vi "FPGA_driver.vi"() -> ()   [LabVIEW 2019]
uses:
  <vilib>/Platform/TimedLoop/XDataNode/timing_clust.ctl
  <vilib>/Platform/TimedLoop/XDataNode/nitl_modes.ctl
  <vilib>/Platform/TimedLoop/XDataNode/wakeup.ctl
  <vilib>/rvi/Emulation/niFpgaGetClockAttributes.vi
  <vilib>/rvi/Emulation/niFpgaSctlEmulationGetInTimedLoop.vi
  <vilib>/rvi/Emulation/niFpgaEmulationReportErrorSimple.vi
  <vilib>/rvi/Emulation/niFpgaProcessEmulError.vi
  <vilib>/rvi/Emulation/niFpgaCriticalErrorInLSC.vi
  <vilib>/rvi/eio/common/nirviEmuTemplateMethod_errors.vi
  <vilib>/rvi/Analysis/common/FxpNativeNode/niFpgaFxpNative.xnode
  <vilib>/eio/EIONode/EIONode.xnode
  <vilib>/platform/TimedLoop/XDataNode/XDataNode.xnode
  <vilib>/Platform/TimedLoop/XDataNode/XDNodeRunTimeDep.lvlib
panel:
  out "Feed Reset":bool
  out "Steer Reset":bool
  in  "Num_cycle_on":u32
  in  "enable?":bool
  out "Encoder Position 2":i16
  in  "Encoder Reload Value 2":i16
  out "clk/pulse":i32
  out "Velocity\nValid?":bool
  in  "Position Ref.":i32
  in  "Num Clocks\nper Period":u32=400000
  in  "Velocity \nLimit":i32=10
  in  "Position Loop\nPeriod (ms)":u32=10
  out "Encoder Position":i16
  in  "Encoder Reload Value":i16
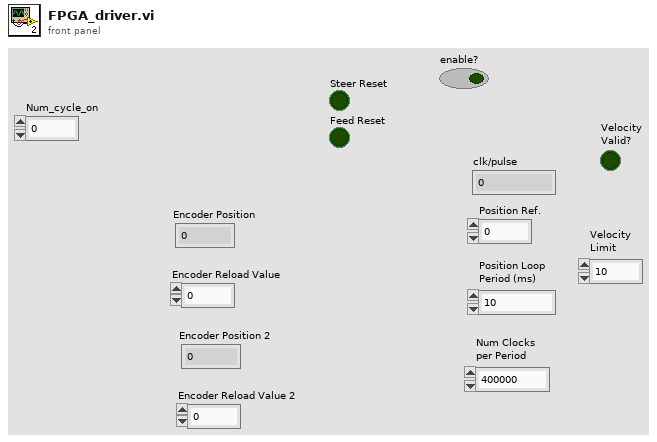
[diagram p1: front panel]
types:
  T1 = typedef "XDNodeRunTimeDep.lvlib/timing_clust.ctl" = cluster{"Expected End [f-1]":u64, "Actual End [f-1]":u64, "Finished Late? [f-1]":bool, "Expected End [i-1]":u64, "Actual End [i-1]":u64, "Finished Late? [i-1]":bool, "Expected Start [i]":u64, "Actual Start [i]":u64, "Expected Start [f]":u64, "Actual Start [f]":u64, "Source Name":string, "Structure Name":string, "Period":i64, "Deadline":i64, "Offset":i64, "Start":i64, "Priority":i32, "Timeout":i32, "Mode":T2, "Wakeup Reason":T3, "Error":errorcluster, "Source Type":string, "Secondary Source Type":string, "Global End Time":u64, "Global Start Time":u64, "Frame Duration":u64, "Iteration Duration":u64, "Assigned CPU":i32, "I/O Scan Engine Mode":u32}
  T2 = typedef "XDNodeRunTimeDep.lvlib/nitl_modes.ctl" = enum32{"No Change", "Process missed periods, maintain original phase", "Discard missed periods, maintain original phase", "Process missed periods, ignore original phase", "Discard missed periods, ignore original phase"}
  T3 = typedef "XDNodeRunTimeDep.lvlib/wakeup.ctl" = enum32{"Normal", "Aborted", "Asynchronous wakeup", "Timing source error", "Timed loop error", "Timeout"}
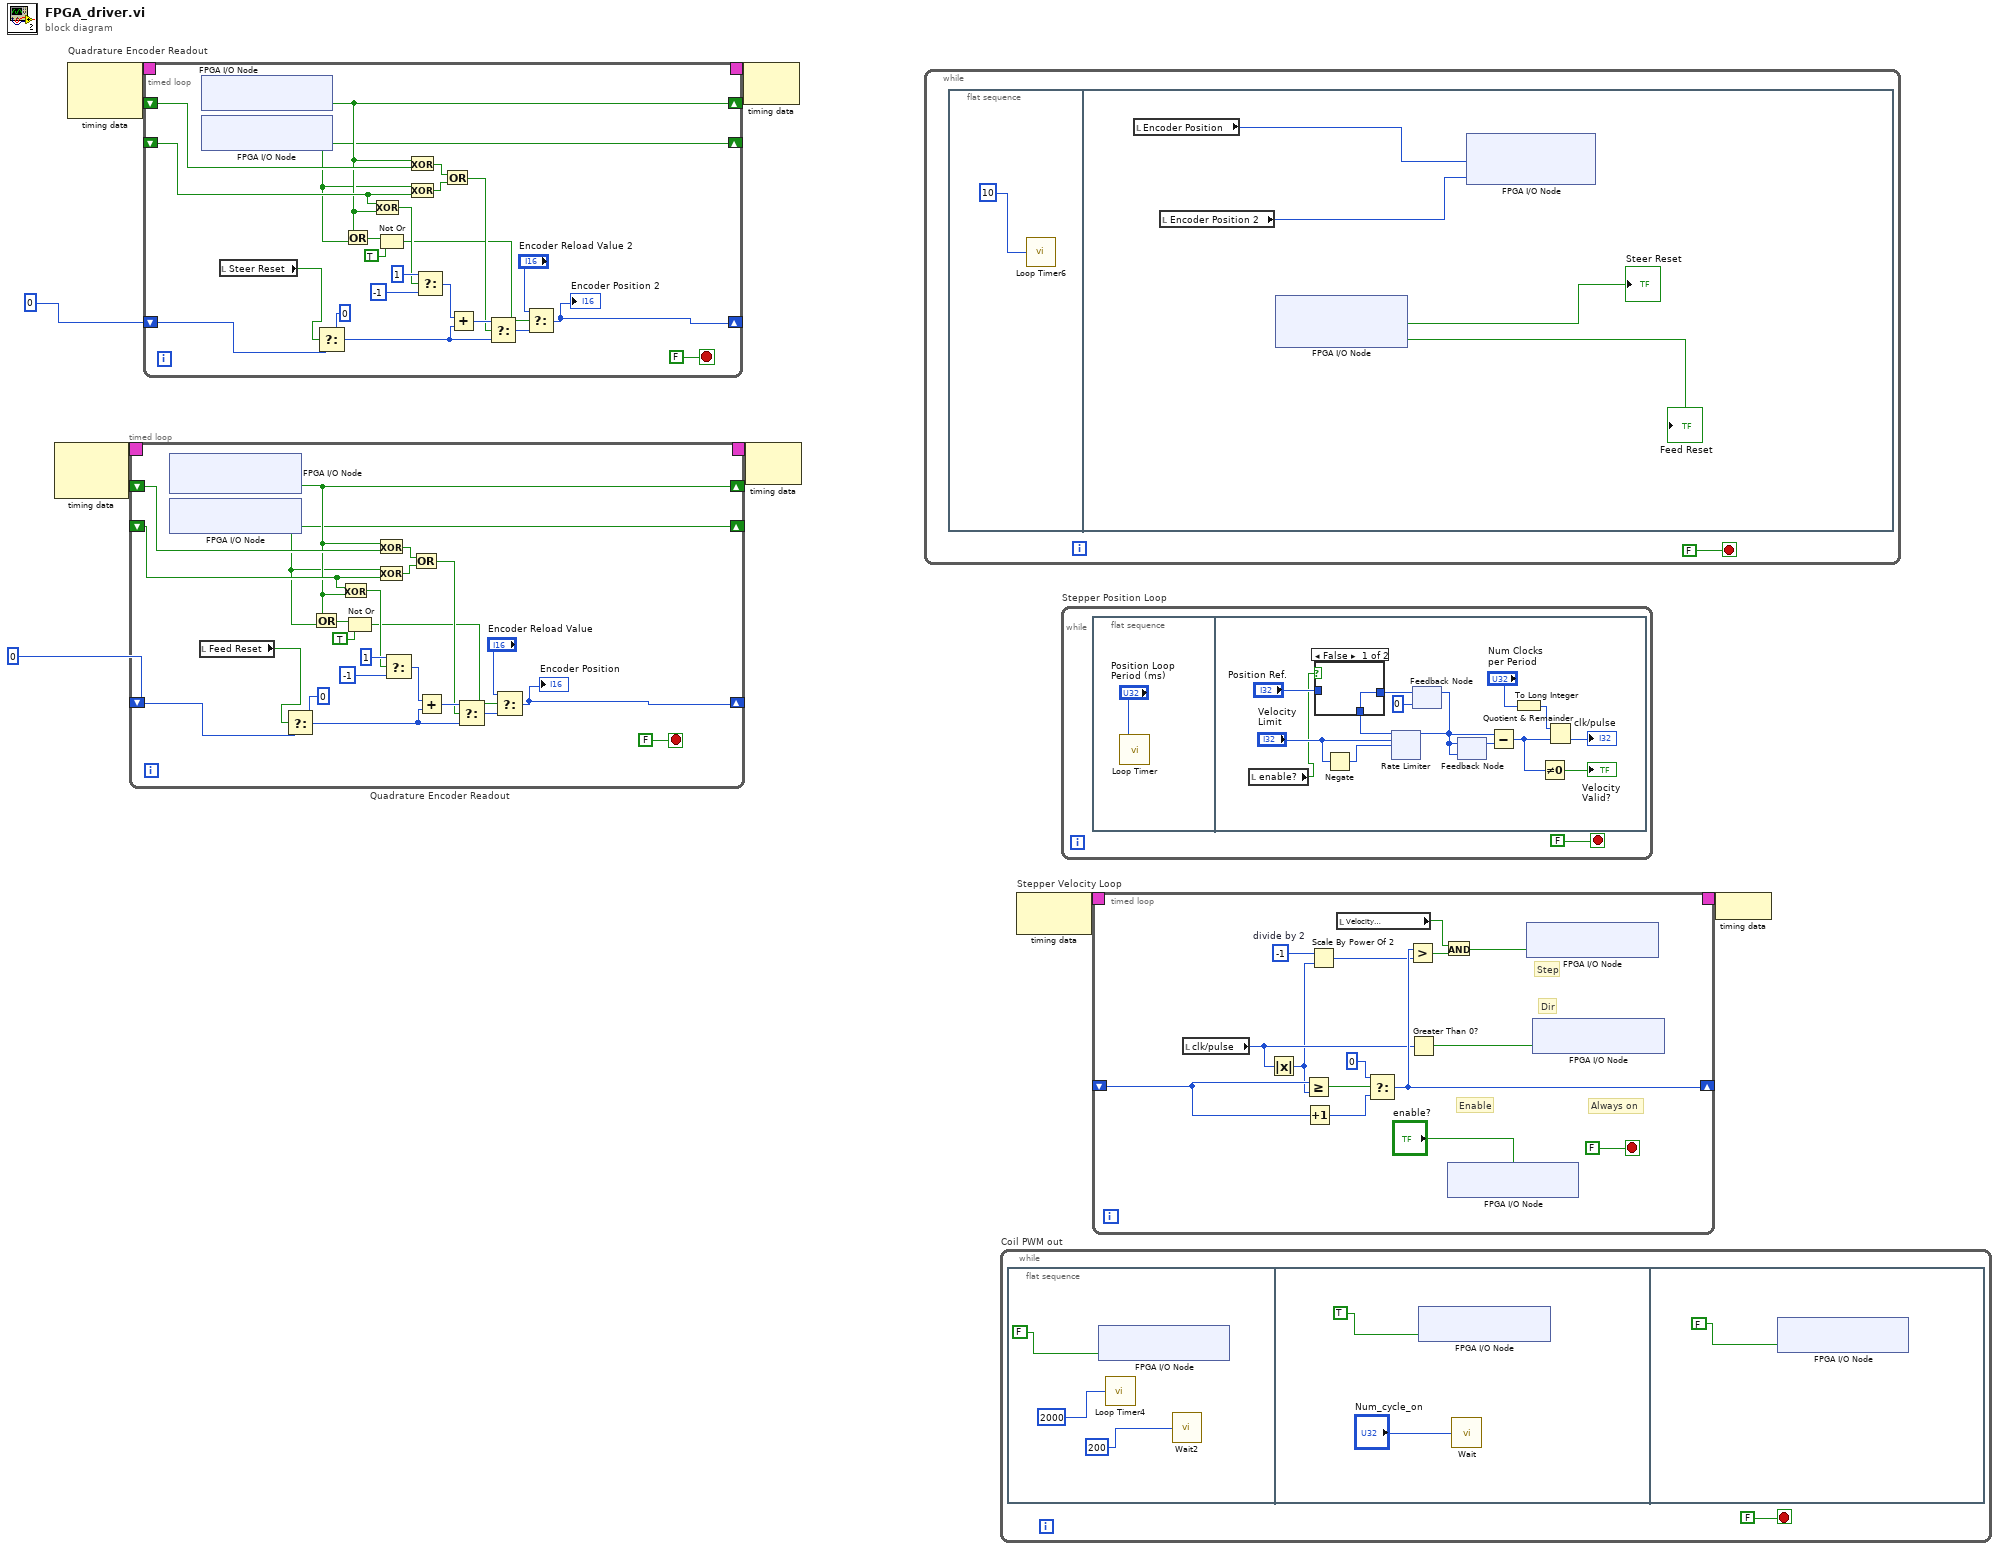
[diagram p0: block diagram]
diagram:
  n1 = node-c288() -> (w8:T1)  [unwired: 2 out]
  n2 = node-c288() -> (w3:T1)  [unwired: 2 out]
  n3 = timed-loop "Quadrature Encoder Readout" {
    timing-out: [_] -> w7
    timing: w8 -> [_]
    shift-left: _ -> [w17]
    shift-right: [w13] -> _
    shift-left: i16 0 -> [w28]
    shift-right: [w10] -> _
    shift-left: _ -> [w18]
    shift-right: [w14] -> _
    stop <- FALSE stop-if-true
    n4 = xnode "FPGA I/O Node"() -> ("ConnectorA/DIO0"=w14:bool)  [unwired: 2 in, 2 out]
    n5 = xnode "FPGA I/O Node"() -> ("ConnectorA/DIO1"=w13:bool)  [unwired: 1 in, 1 out]
    n6 = local read "Feed Reset"() -> (w9:bool)
    n7 = Select(t=i16 0, s=w9, f=w28) -> (s? t:f=w29:i16)
    n8 = Or(x=w14, y=w13) -> (x .or. y?=w12:bool)
    n9 = Exclusive Or(1:w14, 2:w17) -> (0:w19:bool)
    n10 = Not Or(1:TRUE ("y"), 2:w12) -> (0:w16:bool)
    n11 = Exclusive Or(1:w18, 2:w14) -> (0:w21:bool)
    n12 = Exclusive Or(1:w17, 2:w13) -> (0:w22:bool)
    n13 = Select(t=i16 1, s=w19, f=i16 -1) -> (s? t:f=w27:i16)
    n14 = Or(x=w21, y=w22) -> (x .or. y?=w20:bool)
    n15 = Add(x=w27, y=w29) -> (x+y=w31:i16)
    n16 = Select(t=w31, s=w20, f=w29) -> (s? t:f=w24:i16)
    n17 = Select(t="Encoder Reload Value", s=w16, f=w24) -> (s? t:f=w10:i16)
    "Encoder Position" <- w10
  }
  n18 = timed-loop "Quadrature Encoder Readout" {
    timing-out: [_] -> w2
    timing: w3 -> [_]
    shift-left: _ -> [w42]
    shift-right: [w38] -> _
    shift-left: i16 0 -> [w53]
    shift-right: [w35] -> _
    shift-left: _ -> [w43]
    shift-right: [w39] -> _
    stop <- FALSE stop-if-true
    n19 = xnode "FPGA I/O Node"() -> ("ConnectorA/DIO2"=w39:bool)  [unwired: 1 in, 1 out]
    n20 = xnode "FPGA I/O Node"() -> ("ConnectorA/DIO3"=w38:bool)  [unwired: 1 in, 1 out]
    n21 = local read "Steer Reset"() -> (w34:bool)
    n22 = Select(t=i16 0, s=w34, f=w53) -> (s? t:f=w54:i16)
    n23 = Or(x=w39, y=w38) -> (x .or. y?=w37:bool)
    n24 = Exclusive Or(1:w39, 2:w42) -> (0:w44:bool)
    n25 = Not Or(1:TRUE ("y"), 2:w37) -> (0:w41:bool)
    n26 = Exclusive Or(1:w43, 2:w39) -> (0:w46:bool)
    n27 = Exclusive Or(1:w42, 2:w38) -> (0:w47:bool)
    n28 = Select(t=i16 1, s=w44, f=i16 -1) -> (s? t:f=w52:i16)
    n29 = Or(x=w46, y=w47) -> (x .or. y?=w45:bool)
    n30 = Add(x=w52, y=w54) -> (x+y=w56:i16)
    n31 = Select(t=w56, s=w45, f=w54) -> (s? t:f=w49:i16)
    n32 = Select(t="Encoder Reload Value 2", s=w41, f=w49) -> (s? t:f=w35:i16)
    "Encoder Position 2" <- w35
  }
  n33 = node-c288(w2) -> ()  [unwired: 1 out]
  n34 = node-c288(w7) -> ()  [unwired: 1 out]
  n35 = while {
    stop <- FALSE stop-if-true
    n36 = flat-sequence {
      frame #0 {
        n37 = call "Loop Timer6"("Count(mSec)"=u32 10) -> ()  [unwired: 1 out]
      }
      frame #1 {
        n38 = local read "Encoder Position"() -> (w63:i16)
        n39 = local read "Encoder Position 2"() -> (w64:i16)
        n40 = xnode "FPGA I/O Node"() -> ("ConnectorC/DIO6"=→"Steer Reset":bool, "ConnectorC/DIO7"=→"Feed Reset":bool)  [unwired: 2 in, 2 out]
        n41 = xnode "FPGA I/O Node"("ConnectorC/AO0"=w63, "ConnectorC/AO1"=w64) -> ()  [unwired: 2 in, 2 out]
      }
    }
  }
  n42 = while "Coil PWM out" {
    stop <- FALSE stop-if-true
    n43 = flat-sequence {
      frame #0 {
        n44 = xnode "FPGA I/O Node"("ConnectorC/DIO1"=FALSE) -> ()  [unwired: 1 in, 1 out]
        n45 = call "Loop Timer4"("Count(Ticks)"=u32 2000 ("Count(uSec)")) -> ()  [unwired: 1 out]
        n46 = call "Wait2"("Count(Ticks)"=u32 200) -> ()  [unwired: 1 out]
      }
      frame #1 {
        n47 = xnode "FPGA I/O Node"("ConnectorC/DIO1"=TRUE) -> ()  [unwired: 1 in, 1 out]
        n48 = call "Wait"("Count(Ticks)"="Num_cycle_on") -> ()  [unwired: 1 out]
      }
      frame #2 {
        n49 = xnode "FPGA I/O Node"("ConnectorC/DIO1"=FALSE) -> ()  [unwired: 1 in, 1 out]
      }
    }
  }
  n50 = node-c288() -> (w5:T1)  [unwired: 1 in]
  n51 = while "Stepper Position Loop" {
    stop <- FALSE stop-if-true
    n52 = flat-sequence {
      frame #0 {
        n53 = call "Loop Timer"("Count(mSec)"="Position Loop\nPeriod (ms)") -> ()  [unwired: 1 out]
      }
      frame #1 {
        n54 = local read "enable?"() -> (w74:bool)
        n55 = Negate(x="Velocity \nLimit") -> (-x=w81:i32)
        n56 = feedback #1(0 ("output")) -> (w76:i32)
        n57 = case shown="False" w74 {
          tunnel: [w88 w89] -> w79
          tunnel: "Position Ref." -> [_ w89]
          tunnel: w76 -> [w88 _]
          frame False {
          }
          frame True {
          }
        }
        n58 = xnode ("Rate Limiter")("pos slew rate * dt"="Velocity \nLimit", "input"=w79, "neg slew rate * dt"=w81) -> ("output"=w77:i32)  [unwired: 1 in]
        n59 = feedback-in #1(w77) -> ()
        n60 = feedback #2(w77) -> (w86:i32)
        n61 = feedback-in #2(w77) -> ()
        n62 = Subtract(x=w77, y=w86) -> (x-y=w83:i32)
        n63 = To Long Integer(number="Num Clocks\nper Period") -> (32bit integer=w84:i32)
        n64 = Not Equal To 0?(x=w83) -> (x != 0?=→"Velocity\nValid?":bool)
        n65 = Quotient & Remainder(x=w84, y=w83) -> (floor(x/y)=→"clk/pulse":i32)  [unwired: 1 out]
      }
    }
  }
  n66 = timed-loop "Stepper Velocity Loop" {
    timing: w5 -> [_]
    timing-out: [_] -> w4
    shift-right: [w124] -> _
    shift-left: _ -> [w121]
    stop <- FALSE stop-if-true
    w117 = -1  # divide by 2
    # "Always on"
    # "Enable"
    # "Dir"
    # "Step"
    n67 = local read "clk/pulse"() -> (w120:i32)
    n68 = Absolute Value(x=w120) -> (abs(x)=w118:i32)
    n69 = Greater Or Equal?(x=w121, y=w118) -> (x >= y?=w125:bool)
    n70 = Increment(x=w121) -> (x+1=w127:i32)
    n71 = Scale By Power Of 2(n=w117, x=w118) -> (x*2^n=w119:i32)
    n72 = local read "Velocity\nValid?"() -> (w122:bool)
    n73 = Select(t=0, s=w125, f=w127) -> (s? t:f=w124:i32)
    n74 = Greater?(x=w124, y=w119) -> (0:w123:bool)
    n75 = Greater Than 0?(x=w120) -> (x > 0?=w116:bool)
    n76 = And(x=w122, y=w123) -> (x .and. y?=w115:bool)
    n77 = xnode "FPGA I/O Node"("ConnectorC/DIO4"="enable?") -> ()  [unwired: 1 in, 1 out]
    n78 = xnode "FPGA I/O Node"("ConnectorC/DIO2"=w115) -> ()  [unwired: 1 in, 1 out]
    n79 = xnode "FPGA I/O Node"("ConnectorC/DIO3"=w116) -> ()  [unwired: 1 in, 1 out]
  }
  n80 = node-c288(w4) -> ()
